vi "Encoders.vi"(8 "error in (no error)":errorcluster) -> (0 "error out":errorcluster, 1 "Encoder 4":i32, 2 "Encoder 3":i32, 3 "Encoder 2":i32, 5 "Encoder 1":i32)   [LabVIEW 2014]
uses:
  <userlib>/UCSD Robotics Lab/Robotics-Cape/LV/libroboticscape.lvlib
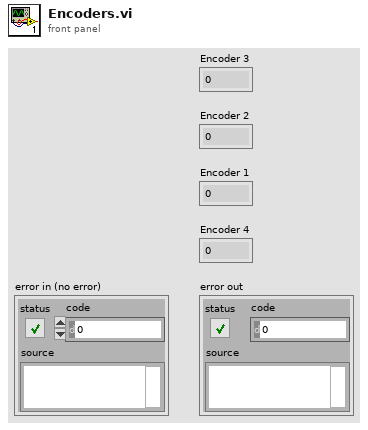
[diagram p1: front panel]
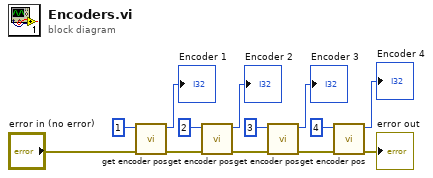
[diagram p0: block diagram]
diagram:
  n1 = call <userlib>:"get encoder pos.vi"("error in (no error)"="error in (no error)", "ch"=1) -> ("error out"=w2:errorcluster, "function return"=→"Encoder 1":i32)  [unwired: 8 in]
  n2 = call <userlib>:"get encoder pos.vi"("error in (no error)"=w2, "ch"=2) -> ("error out"=w3:errorcluster, "function return"=→"Encoder 2":i32)  [unwired: 8 in]
  n3 = call <userlib>:"get encoder pos.vi"("error in (no error)"=w3, "ch"=3) -> ("error out"=w4:errorcluster, "function return"=→"Encoder 3":i32)  [unwired: 8 in]
  n4 = call <userlib>:"get encoder pos.vi"("error in (no error)"=w4, "ch"=4) -> ("error out"=→"error out":errorcluster, "function return"=→"Encoder 4":i32)  [unwired: 8 in]
